vi "Control Panel Values Changed.vi"(8 "error in (no error)":errorcluster, 9 "Old value":variant, 10 "New value":variant, 11 "Test Class in":refnum<class "Test Class.lvclass">) -> (0 "error out":errorcluster, 3 "Test Class out":refnum<class "Test Class.lvclass">)   [LabVIEW 2015, in "Test Class.lvclass"]
uses:
  Test Class.lvclass
  Test FP data.ctl
  Device/Device.lvclass
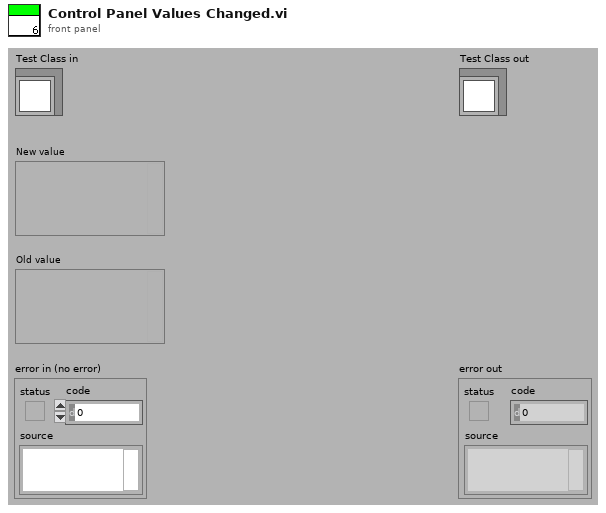
[diagram p1: front panel]
types:
  T1 = typedef "Test FP data.ctl" = cluster{"Channels to scan":i32[], "Scan settling, s":dbl, "Read temperature":bool, "Read heater":bool, "Control Instrument":bool, "Set point":dbl, "Heater Range":enum16{"Off", "31.6uA", "100uA", "316uA", "1mA", "3.16uA", "31.6mA", "100mA", "10mA"}, "Test":dbl}
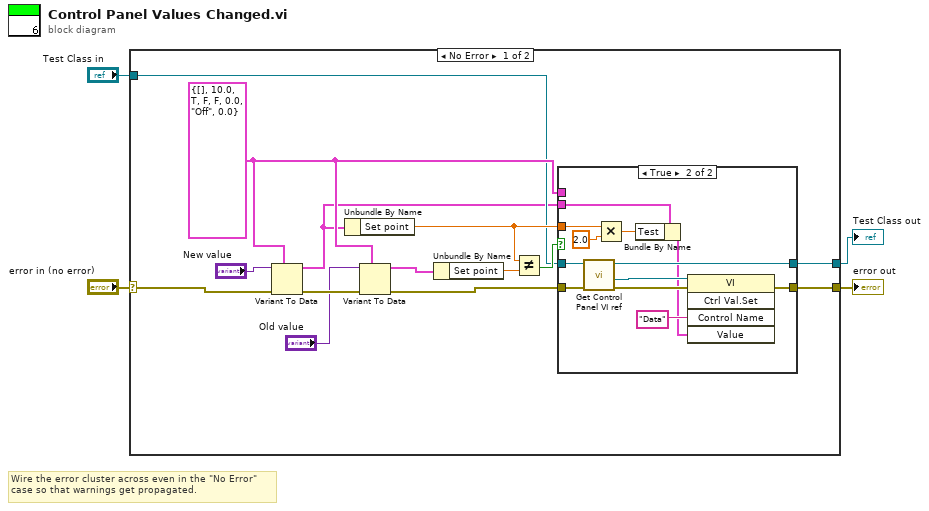
[diagram p0: block diagram]
diagram:
  # "Wire the error cluster across even in the \"No Error\"\ncase so that warnings get propagated."
  n1 = case shown="No Error" "error in (no error)" {
    selector: "error in (no error)" -> [w17 w34]
    tunnel: [w10 w34] -> w3
    tunnel: [w6 w33] -> w1
    tunnel: "Test Class in" -> [w7 w33]
    frame No Error {
      w9 = T1 {"Channels to scan"=[], "Scan settling, s"=10.0, "Read temperature"=TRUE, "Read heater"=FALSE, "Control Instrument"=FALSE, "Set point"=0.0, "Heater Range"=enum."Off", "Test"=0.0} ("Data")
      n2 = Variant To Data(error in=w17, type=w9, Variant="New value") -> (data=w5:T1, error out=w16:errorcluster)
      n3 = Unbundle By Name(w5) -> ("Set point"=w8:dbl)
      n4 = Variant To Data(error in=w16, type=w9, Variant="Old value") -> (data=w14:T1, error out=w11:errorcluster)
      n5 = Unbundle By Name(w14) -> ("Set point"=w13:dbl)
      n6 = Not Equal?(x=w8, y=w13) -> (x != y?=w12:bool)
      n7 = case shown="True" w12 {
        tunnel: w11 -> [w19 w28]
        tunnel: [w19 w24] -> w10
        tunnel: w7 -> [w20 w26]
        tunnel: w9 -> [_ _]
        tunnel: w8 -> [_ w32]
        tunnel: [w20 w23] -> w6
        tunnel: w5 -> [_ w22]
        frame False {
        }
        frame True {
          n8 = call "Get Control Panel VI ref.vi"("error in (no error)"=w28, "Device in"=w26) -> ("error out"=w27:errorcluster, "vi ref out"=w25:refnum<vi>, "Device out"=w23:refnum<class "Test Class.lvclass">)  [unwired: 7 in]
          n9 = Multiply(x=w32, y=2.0) -> (x*y=w30:dbl)
          n10 = Bundle By Name(cluster=w22, "Test"=w30) -> (w21:T1)
          n11 = invoke class="VI" method="Ctrl Val.Set"(reference=w25, error in=w27, "Control Name"="Data", "Value"=w21) -> (error out=w24:errorcluster)  [unwired: 1 in, 4 out]
        }
      }
    }
    frame Error {
    }
  }
  "error out" <- w3
  "Test Class out" <- w1
